vi "d0630view.vi"(8 "error in":errorcluster) -> (0 "error out":errorcluster, 10 "Y2":dbl, 11 "X2":dbl)   [LabVIEW 2019]
panel:
  out "Xmin":dbl
  out "x1":dbl
  out "Ymin":dbl
  out "y1":dbl
  out "Image Out 2":T1(plugin-control)
  out "subarray":dbl[](array[numeric])
  out "Number of Particles (Particle Analysis 1)":i32
  in  "Stop (F)":bool
  out "Image Out":T1(plugin-control)
  out "Particle Measurements (Pixels) (Particle Analysis 1)":dbl[][](array[numeric]) format="%.2f"
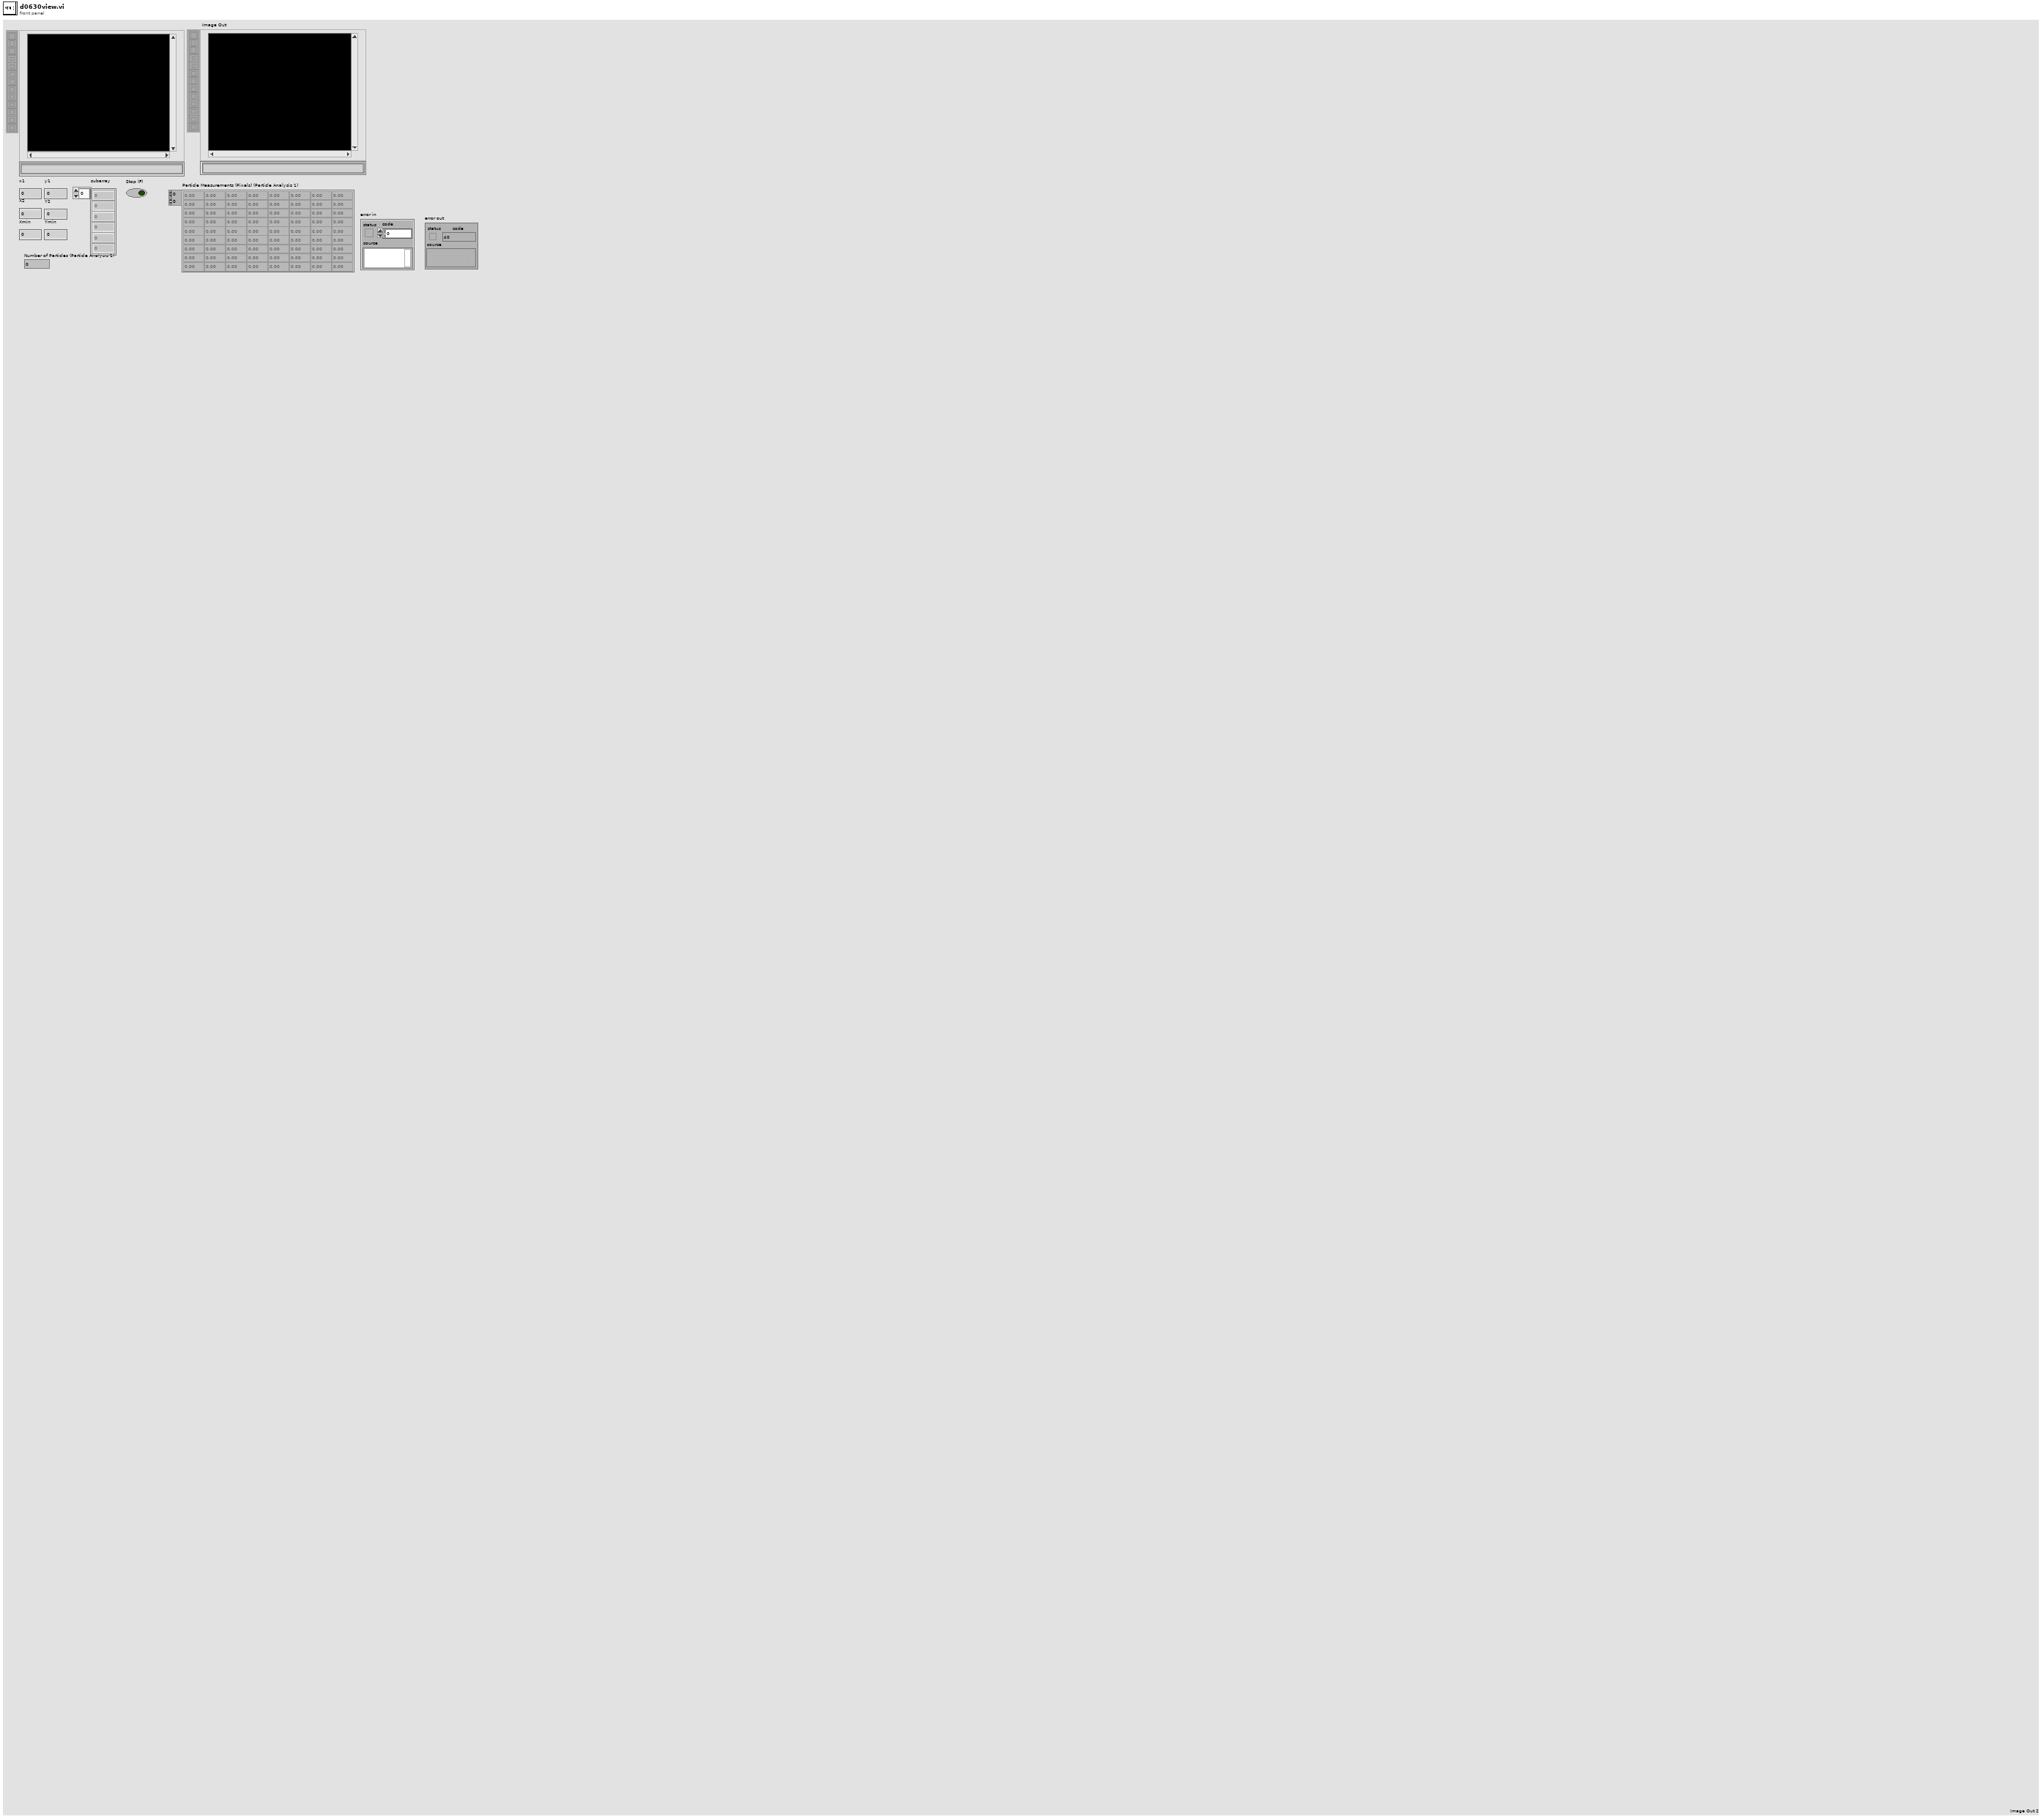
[diagram p1: front panel]
types:
  T1 = typedef "IMAQ Image.ctl" = refnum<image>
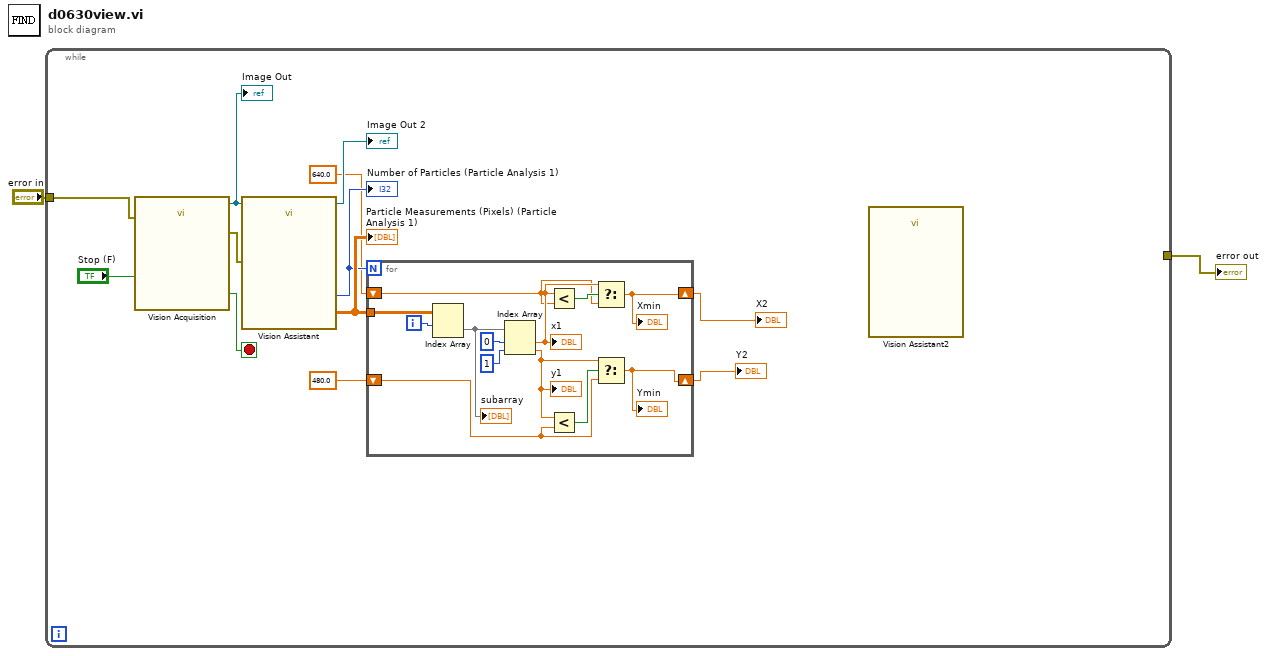
[diagram p0: block diagram]
diagram:
  n1 = while {
    tunnel: [_] -> w2
    tunnel: "error in" -> [w5]
    stop <- w13 stop-if-true
    n2 = call "Vision Acquisition"("Stop (F)"="Stop (F)", "error in"=w5) -> ("Image Out"=w12:T1, "Stopped"=w13:bool, "error out"=w6:errorcluster)  [unwired: 23 in]
    "Image Out" <- w12
    n3 = call "Vision Assistant"("Image In"=w12, "error in"=w6) -> ("Image Out"=→"Image Out 2":T1, "Number of Particles (Particle Analysis 1)"=w9:i32, "Particle Measurements (Pixels) (Particle Analysis 1)"=w10:dbl[][])  [unwired: 22 in, 1 out]
    "Particle Measurements (Pixels) (Particle Analysis 1)" <- w10
    "Number of Particles (Particle Analysis 1)" <- w9
    n4 = for {
      N: w9 -> [_]
      tunnel: w10 -> [w26]
      shift-right: [w20] -> w3
      shift-left: 480.0 -> [w21]
      shift-right: [w16] -> w4
      shift-left: 640.0 ("Numeric") -> [w15]
      i -> [w25]
      n5 = Index Array(array=w26, index (row)=w25) -> (element=w27:dbl[])  [unwired: 1 in]
      "subarray" <- w27
      n6 = Index Array(array=w27, index #1=0 ("index"), index #2=1 ("index")) -> (element #1=w17:dbl, element #2=w19:dbl)
      "y1" <- w19
      "x1" <- w17
      n7 = Less?(x=w17, y=w15) -> (x < y?=w18:bool)
      n8 = Less?(x=w19, y=w21) -> (x < y?=w22:bool)
      n9 = Select(t=w17, s=w18, f=w15) -> (s? t:f=w16:dbl)
      "Xmin" <- w16
      n10 = Select(t=w19, s=w22, f=w21) -> (s? t:f=w20:dbl)
      "Ymin" <- w20
    }
    "X2" <- w4
    "Y2" <- w3
    n11 = call "Vision Assistant2"() -> ()  [unwired: 25 in, 3 out]
  }
  "error out" <- w2
